vi "BurstModeCompleteRoutedMessage_Parse.vi"(8 "error in (no error)":errorcluster, 11 "message":variant) -> (0 "error out":errorcluster, 2 "BurstModeComplete":T1)   [LabVIEW 2017, in "BurstMode.lvlib"]
uses:
  <vilib>/addons/InsightCM/Devices/Shared/Cms/CmsBurstMode/BurstMode.lvlib
  <vilib>/addons/InsightCM/Devices/Shared/Cms/CmsBurstMode/controls/BurstModeComplete.ctl
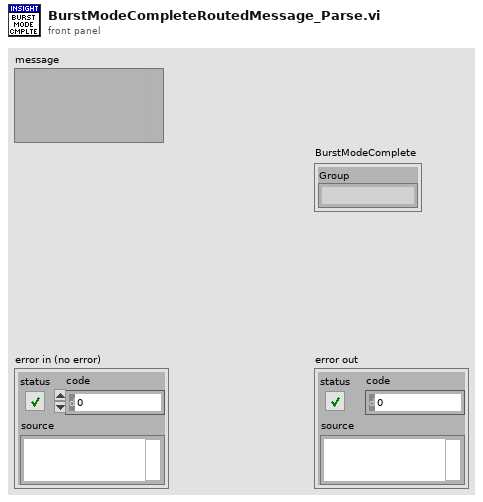
[diagram p1: front panel]
types:
  T1 = typedef "BurstMode.lvlib/BurstModeComplete.ctl" = cluster{"Group":string}
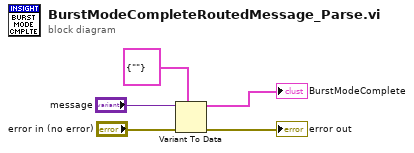
[diagram p0: block diagram]
diagram:
  n1 = Variant To Data(error in="error in (no error)", type=T1 {"Group"=""} ("BurstModeComplete"), Variant="message") -> (data=→"BurstModeComplete":T1, error out=→"error out":errorcluster)
